vi "isRunning.vi"(8 "error in (no error)":errorcluster, 11 "StaticOutputEditor in":refnum<class "StaticOutputEditor.lvclass">) -> (0 "error out":errorcluster, 2 "running?":bool, 3 "StaticOutputEditor out":refnum<class "StaticOutputEditor.lvclass">)   [LabVIEW 2009, in "Views.lvlib" / "ScriptEditor.lvlib" / "StaticOutputEditor.lvclass"]
uses:
  StaticOutputEditor.lvclass
  StaticOutputEditor.lvclass/StaticOutputEditor.ctl
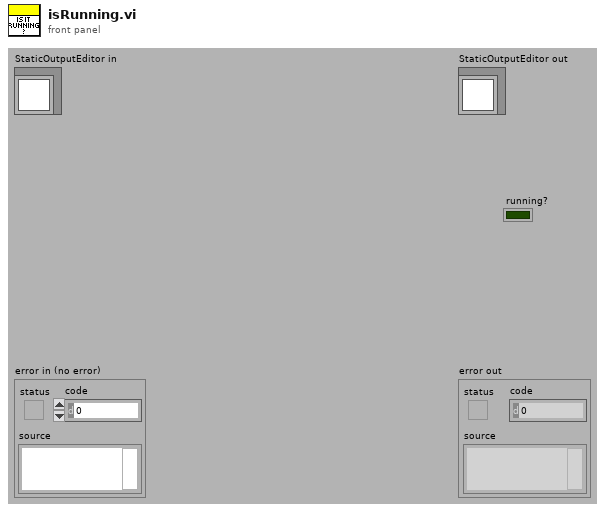
[diagram p1: front panel]
types:
  T1 = enum32{"Bad", "Idle", "Run top level", "Running"}
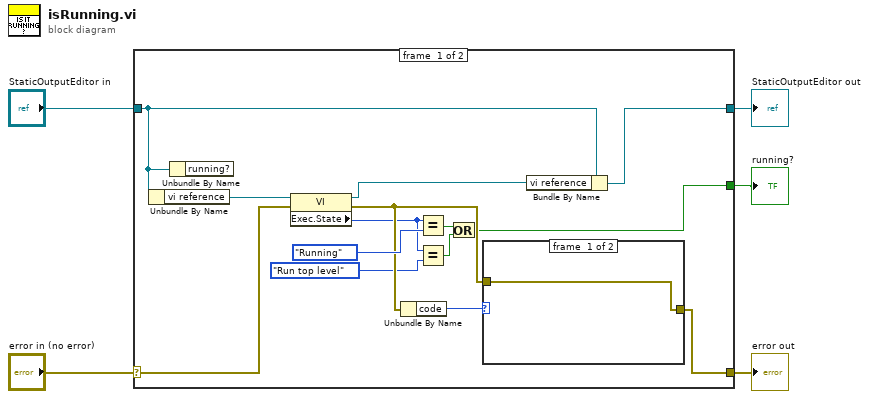
[diagram p0: block diagram]
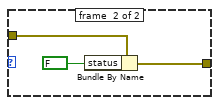
[diagram p2: hidden frame]
diagram:
  n1 = case shown="No Error" "error in (no error)" {
    selector: "error in (no error)" -> [w17 w25]
    tunnel: [w11 w25] -> w4
    tunnel: [w14 w24] -> w2
    tunnel: "StaticOutputEditor in" -> [w15 w24]
    tunnel: [w6 _] -> w1
    frame #0 {
      n2 = Unbundle By Name(w15) -> ("vi reference"=w19:refnum<vi>)
      n3 = Unbundle By Name(w15) -> ()  [unwired: 1 out]
      n4 = property class="VI"(reference=w19, error in=w17) -> (reference out=w16:refnum<vi>, error out=w12:errorcluster, "Exec.State"=w10:T1)
      n5 = Unbundle By Name(w12) -> ("code"=w13:i32)
      n6 = Equal?(x=w10, y=T1."Running" ("Execution:State")) -> (x = y?=w8:bool)
      n7 = Equal?(x=w10, y=T1."Run top level" ("Execution:State")) -> (x = y?=w7:bool)
      n8 = Or(x=w8, y=w7) -> (x .or. y?=w6:bool)
      n9 = case shown="1026" w13 {
        tunnel: w12 -> [w20 w23]
        tunnel: [w20 w22] -> w11
        frame #0 {
        }
        frame #1 {
          n10 = Bundle By Name(cluster=w23, "status"=FALSE) -> (w22:errorcluster)
        }
      }
      n11 = Bundle By Name(cluster=w15, "vi reference"=w16) -> (w14:refnum<class "StaticOutputEditor.lvclass">)
    }
    frame #1 {
    }
  }
  "error out" <- w4
  "StaticOutputEditor out" <- w2
  "running?" <- w1
